vi "Asylum_Driver_GoToInitialPoint.vi"(8 "error in (no error)":errorcluster, 9 "Z Setpoint":dbl, 10 "Coordinate":cluster{"X":dbl, "Y":dbl, "Speed":dbl}, 11 "Application":refnum<k7>) -> (0 "error out":errorcluster, 3 "Application":refnum<k7>)   [LabVIEW 2020]
uses:
  Asylum_Driver_XYMetersToVoltage.vi
  <vilib>/Levylab/Asylum AFM API/Igor Data/LVArraytoIgorWave/NumericArraytoIgorWave.vi
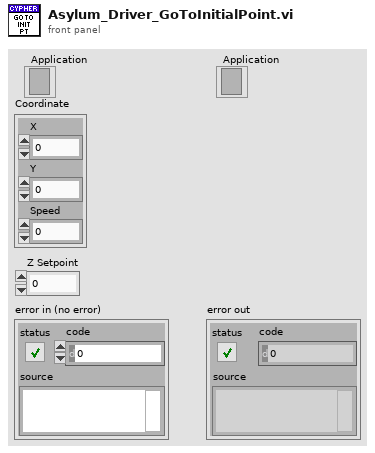
[diagram p1: front panel]
types:
  T1 = cluster{"setpoint":dbl, "pgain":dbl, "igain":dbl, "sgain":dbl}
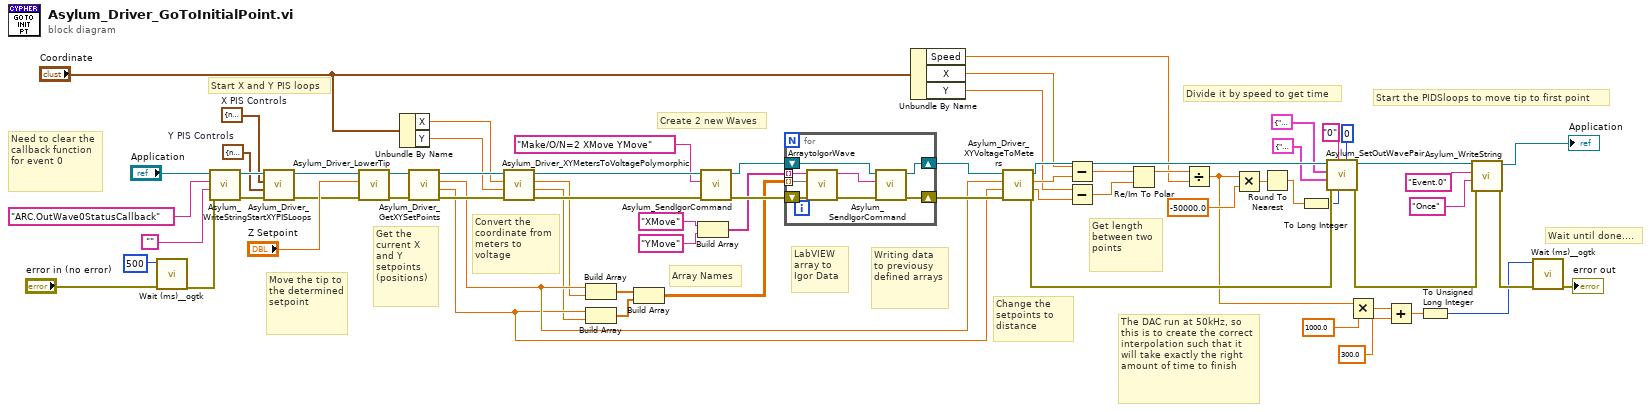
[diagram p0: block diagram]
diagram:
  w11 = T1 {"setpoint"=nan, "pgain"=0.0, "igain"=61660.0, "sgain"=0.0}  # Y PIS Controls
  w12 = T1 {"setpoint"=nan, "pgain"=0.0, "igain"=-63096.0, "sgain"=0.0}  # X PIS Controls
  # "Wait until done...."
  # "Start the PIDSloops to move tip to first point"
  # "The DAC run at 50kHz, so this is to create the correct interpolation such that it will take exactly the right amount of time to finish"
  # "Divide it by speed to get time"
  # "Get length between two points"
  # "Change the setpoints to distance"
  # "Array Names"
  # "Writing data to previousy defined arrays"
  # "LabVIEW array to Igor Data"
  # "Create 2 new Waves"
  # "Convert the coordinate from meters to voltage"
  # "Get the current X and Y setpoints (positions)"
  # "Move the tip to the determined setpoint"
  # "Start X and Y PIS loops"
  # "Need to clear the callback function for event 0"
  n1 = call <userlib>:"Wait (ms)__ogtk.vi"("error in (no error)"="error in (no error)", "milliseconds to wait"=u32 500) -> ("error out"=w61:errorcluster)  [unwired: 8 in, 1 out]
  n2 = call <vilib>:"Asylum_WriteString.vi"("error in (no error)"=w61, "valueString"="", "parameterName"="ARC.OutWave0StatusCallback", "Application"="Application") -> ("error out"=w55:errorcluster, "Application"=w64:refnum<k7>)  [unwired: 6 in]
  n3 = call "Asylum_Driver_StartXYPISLoops.vi"("error in (no error)"=w55, "Y PIS Controls"=w11, "X PIS Controls"=w12, "Application"=w64) -> ("error out"=w56:errorcluster, "Application"=w63:refnum<k7>)  [unwired: 6 in]
  n4 = call "Asylum_Driver_LowerTip.vi"("error in (no error)"=w56, "Z Setpoint"="Z Setpoint", "Application"=w63) -> ("error out"=w57:errorcluster, "Application"=w62:refnum<k7>)  [unwired: 7 in]
  n5 = Unbundle By Name("Coordinate") -> ("X"=w14:dbl, "Y"=w17:dbl)
  n6 = call "Asylum_Driver_GetXYSetPoints.vi"("error in (no error)"=w57, "Application"=w62) -> ("error out"=w42:errorcluster, "Y Setpoint"=w6:dbl, "X Setpoint"=w8:dbl, "Application"=w58:refnum<k7>)  [unwired: 6 in]
  n7 = call-poly "Asylum_Driver_XYMetersToVoltagePolymorphic.vi"("error in (no error)"=w42, "Y Coordinate"=w17, "X Coordinate"=w14, "Application"=w58) -> ("error out"=w53:errorcluster, "Y Voltage"=w5:dbl, "X Voltage"=w7:dbl, "Application"=w54:refnum<k7>)  [unwired: 4 in]
  n8 = Build Array(w8, w7) -> (w51:dbl[])
  n9 = Build Array(w6, w5) -> (w50:dbl[])
  n10 = Build Array(w51, w50) -> (w45:dbl[][])
  n11 = Build Array("XMove", "YMove") -> (w46:string[])
  n12 = call <vilib>:"Asylum_SendIgorCommand.vi"("error in (no error)"=w53, "command"="Make/O/N=2 XMove YMove", "Application"=w54) -> ("error out"=w47:errorcluster, "Application"=w44:refnum<k7>)  [unwired: 5 in, 2 out]
  n13 = for {
    tunnel: w46 -> [w74] mode=indexing
    tunnel: w45 -> [w73] mode=indexing
    shift-right: [w71] -> w41
    shift-left: w44 -> [w72]
    shift-right: [w70] -> w43
    shift-left: w47 -> [w76]
    n14 = call-poly <vilib>:"ArraytoIgorWave.vi"("error in (no error)"=w76, "Wave"=w73, "Name"=w74) -> ("error out"=w75:errorcluster, "Igor Wave"=w69:string)  [unwired: 7 in]
    n15 = call <vilib>:"Asylum_SendIgorCommand.vi"("error in (no error)"=w75, "command"=w69, "Application"=w72) -> ("error out"=w70:errorcluster, "Application"=w71:refnum<k7>)  [unwired: 5 in, 2 out]
  }
  n16 = Unbundle By Name("Coordinate") -> ("Speed"=w15:dbl, "X"=w18:dbl, "Y"=w16:dbl)
  n17 = call "Asylum_Driver_XYVoltageToMeters.vi"("error in (no error)"=w43, "Y Voltage"=w6, "X Voltage"=w8, "Application"=w41) -> ("error out"=w34:errorcluster, "Y Meters"=w39:dbl, "X Meters"=w40:dbl, "Application"=w31:refnum<k7>)  [unwired: 4 in]
  n18 = Subtract(x=w18, y=w40) -> (x-y=w38:dbl)
  n19 = Subtract(x=w16, y=w39) -> (x-y=w37:dbl)
  n20 = Re/Im To Polar(2:w37, 3:w38) -> (1:w36:dbl)  [unwired: 1 out]
  n21 = Divide(x=w36, y=w15) -> (x/y=w10:dbl)
  n22 = Multiply(x=w10, y=-50000.0) -> (x*y=w21:dbl)
  n23 = Round To Nearest(number=w21) -> (nearest integer value=w2:dbl)
  n24 = To Long Integer(number=w2) -> (32bit integer=w1:i32)
  n25 = call <vilib>:"Asylum_SetOutWavePair.vi"("whichBank"=0, "interpolation"=w1, "eventString"="0", "error in (no error)"=w34, "Wave B"=cluster{"channelStringB":string, "waveB":string} {"channelStringB"="PIDSLoop.1.Setpoint", "waveB"="YMove"}, "Wave A"=cluster{"channelStringA":string, "waveA":string} {"channelStringA"="PIDSLoop.0.Setpoint", "waveA"="XMove"}, "Application"=w31) -> ("error out"=w26:errorcluster, "Application"=w28:refnum<k7>)  [unwired: 3 in]
  n26 = Multiply(x=w10, y=1000.0) -> (x*y=w23:dbl)
  n27 = Add(x=w23, y=300.0) -> (x+y=w4:dbl)
  n28 = To Unsigned Long Integer(number=w4) -> (unsigned 32bit integer=w3:u32)
  n29 = call <vilib>:"Asylum_WriteString.vi"("error in (no error)"=w26, "valueString"="Once", "parameterName"="Event.0", "Application"=w28) -> ("error out"=w20:errorcluster, "Application"=→"Application":refnum<k7>)  [unwired: 6 in]
  n30 = call <userlib>:"Wait (ms)__ogtk.vi"("error in (no error)"=w20, "milliseconds to wait"=w3) -> ("error out"=→"error out":errorcluster)  [unwired: 8 in, 1 out]
